vi "TODO.vi"   [LabVIEW 2024, in "Utilities.lvlib"]
uses:
  Utilities.lvlib
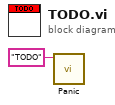
[diagram p0: block diagram]
diagram:
  n1 = call "Panic.vi"("message (\"\")"="TODO" ("message (\"\")")) -> ()  [unwired: 11 in]
